vi "停止采集(M).vi"(8 "错误输入":errorcluster caption="错误输入（无错误）", 11 "设备句柄入":i32) -> (0 "错误输出":errorcluster, 3 "设备句柄":i32=1)   [LabVIEW 2016]
uses:
  dll/em9636.dll
panel:
  in  "超时毫秒":i32=1000
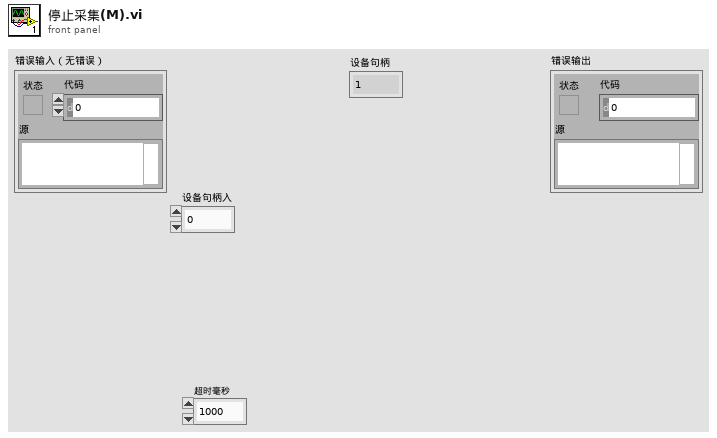
[diagram p1: front panel]
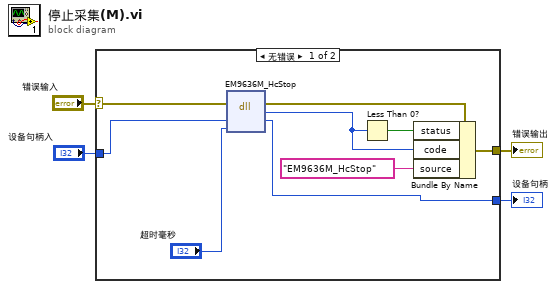
[diagram p0: block diagram]
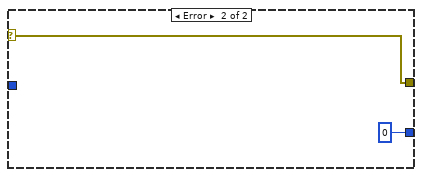
[diagram p2: hidden frame]
diagram:
  n1 = case shown="无错误" "错误输入" {
    selector: "错误输入" -> [w13 w15]
    tunnel: [w9 w15] -> w3
    tunnel: [w5 0 ("错误")] -> w2
    tunnel: "设备句柄入" -> [w7 _]
    frame No Error {
      n2 = dll-call lib="PTH2kabs CUsers\nAdministratorDesktopEM9636*EM9636系列_demo_labview(调用DLL方式)dll\nem9636.dll" fn="EM9636M_HcStop"(error in=w13, "设备句柄"=w7, "超时毫秒"="超时毫秒") -> (error out=w11:errorcluster, "错误"=w8:i32, "设备句柄"=w5:i32)  [unwired: 3 in, 1 out]
      n3 = Less Than 0?(x=w8) -> (x < 0?=w10:bool)
      n4 = Bundle By Name(cluster=w11, "status"=w10, "code"=w8, "source"="EM9636M_HcStop") -> (w9:errorcluster)
    }
    frame Error {
    }
  }
  "错误输出" <- w3
  "设备句柄" <- w2
